vi "CenterPoint.vi"(8 "error in (no error)":errorcluster, 11 "Losange in":refnum<class "Losange.lvclass">) -> (0 "error out":errorcluster, 2 "CenterPoint":refnum<class "Point.lvclass">, 3 "Losange out":refnum<class "Losange.lvclass">)   [LabVIEW 2021, in "Picture2D.lvlib" / "Losange.lvclass"]
uses:
  Losange.lvclass
  Point/Point.lvclass
  Losange.lvclass/Losange.ctl
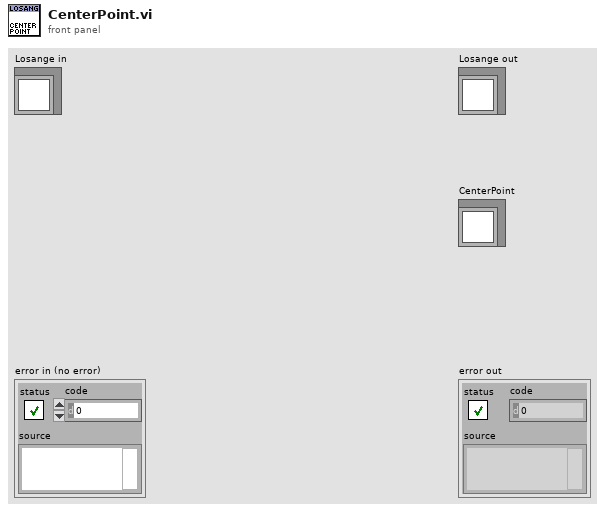
[diagram p1: front panel]
types:
  T1 = cluster{"left":i16, "top":i16, "right":i16, "bottom":i16}
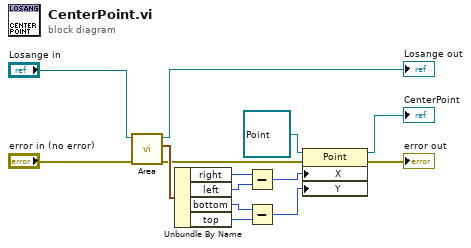
[diagram p0: block diagram]
diagram:
  n1 = call-dynamic "Area.vi"("error in (no error)"="error in (no error)", "Triangle in"="Losange in") -> ("error out"=w2:errorcluster, "rect"=w12:T1, "Triangle out"=→"Losange out":refnum<class "Losange.lvclass">)  [unwired: 7 in]
  n2 = Unbundle By Name(w12) -> ("right"=w11:i16, "left"=w10:i16, "bottom"=w9:i16, "top"=w8:i16)
  n3 = Subtract(x=w11, y=w10) -> (x-y=w5:i16)
  n4 = Subtract(x=w9, y=w8) -> (x-y=w4:i16)
  n5 = property class="Point"(reference=refnum<class "Point.lvclass"> refnum ("CenterPoint"), error in=w2, "X"=w5, "Y"=w4) -> (reference out=→"CenterPoint":refnum<class "Point.lvclass">, error out=→"error out":errorcluster)
